vi "Insight_R_Total_Pts.vi"(8 "error in (no error)":errorcluster, 11 "telnet connection":T1) -> (0 "error out":errorcluster, 1 "response data":string, 2 "Total Points":u32, 3 "telnet  connection out":T1)   [LabVIEW 2014]
doc: "Insight Photonic Solutions\n\nThis VI reads the Total Number of Points in the sweep of the laser, including the Valid and Invalid points.\n\nver 2.0 - updated command syntax\nver 2.1 - return full response string and detect unrecognized command or parameters\nver 3.2 - modify parser to accept responses from Atlas version 3.1 and earlier or version 3.2 and later."
uses:
  Telnet Session.ctl
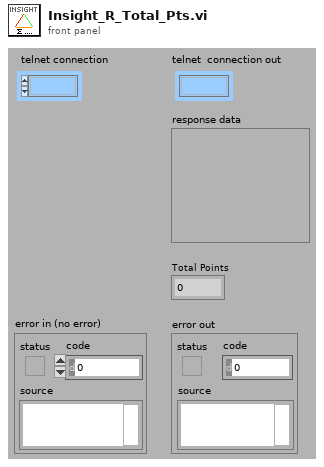
[diagram p1: front panel]
types:
  T1 = typedef "Telnet Session.ctl" = refnum<k1>
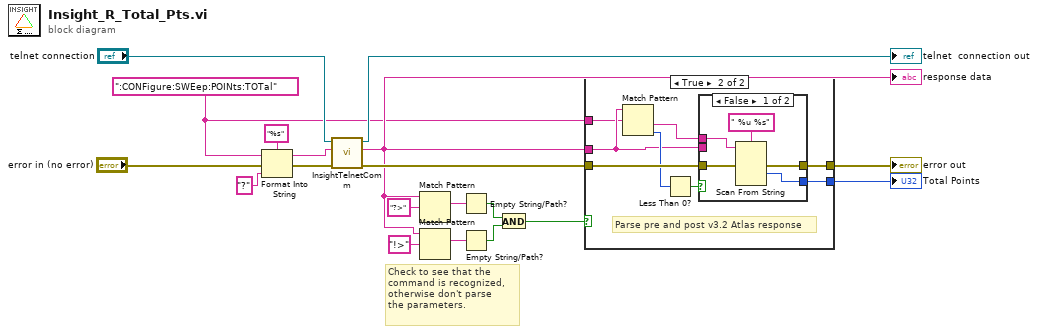
[diagram p0: block diagram]
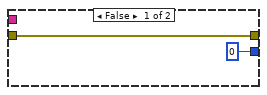
[diagram p2: hidden frame]
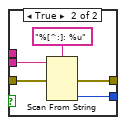
[diagram p3: hidden frame]
diagram:
  w2 = ":CONFigure:SWEep:POINts:TOTal" ("String")
  # "Check to see that the \ncommand is recognized,\notherwise don't parse \nthe parameters."
  n1 = Format Into String(format string="%s", initial string=w2, error in="error in (no error)", "?" ("input 1")) -> (resulting string=w5:string, error out=w6:errorcluster)
  n2 = call "InsightTelnetComm.vi"("error in"=w6, "write buffer (\"\")"=w5, "telnet connection"="telnet connection") -> ("error out"=w10:errorcluster, "response data"=w9:string, "telnet  connection out"=→"telnet  connection out":T1)  [unwired: 4 in]
  "response data" <- w9
  n3 = Match Pattern(string=w9, regular expression="?>") -> (match substring=w16:string)  [unwired: 1 in, 3 out]
  n4 = Match Pattern(string=w9, regular expression="!>") -> (match substring=w15:string)  [unwired: 1 in, 3 out]
  n5 = Empty String/Path?(string/path=w16) -> (empty?=w13:bool)
  n6 = Empty String/Path?(string/path=w15) -> (empty?=w12:bool)
  n7 = And(x=w13, y=w12) -> (x .and. y?=w1:bool)
  n8 = case shown="True" w1 {
    tunnel: [w21 w27] -> w11
    tunnel: w10 -> [w21 w26]
    tunnel: w9 -> [_ w23]
    tunnel: [u32 0 ("default value 1") w28] -> w8
    tunnel: w2 -> [_ w22]
    frame False {
    }
    frame True {
      # "Parse pre and post v3.2 Atlas response"
      n9 = Match Pattern(string=w23, regular expression=w22) -> (after substring=w24:string, offset past match=w25:i32)  [unwired: 1 in, 2 out]
      n10 = Less Than 0?(x=w25) -> (x < 0?=w29:bool)
      n11 = case shown="False" w29 {
        tunnel: w24 -> [w33 _]
        tunnel: w23 -> [_ w38]
        tunnel: [w34 w39] -> w27
        tunnel: [w31 w36] -> w28
        tunnel: w26 -> [w30 w35]
        frame False {
          n12 = Scan From String(format string=" %u %s" ("f"), input string=w33, error in=w30) -> (error out=w34:errorcluster, output 1=w31:u32)  [unwired: 4 in, 2 out]
        }
        frame True {
          n13 = Scan From String(format string="%[^:]: %u", input string=w38, error in=w35) -> (error out=w39:errorcluster, output 2=w36:u32)  [unwired: 4 in, 2 out]
        }
      }
    }
  }
  "error out" <- w11
  "Total Points" <- w8
